vi "ShoulderGetPosition.vi"() -> (0 "SholdrPosDeg":dbl)   [LabVIEW 2023]
uses:
  Elevator/ElevatorGlobal.vi
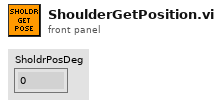
[diagram p1: front panel]
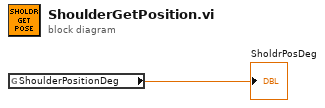
[diagram p0: block diagram]
diagram:
  n1 = global read "ElevatorGlobal.vi" "ShoulderPositionDeg"() -> (→"SholdrPosDeg":dbl)
